vi "Calculate Built Version.vi"(0 "Installer_LV in":refnum<class "Installer_LV.lvclass">, 11 "error in (no error)":errorcluster) -> (4 "Installer_LV out":refnum<class "Installer_LV.lvclass">, 15 "error out":errorcluster)   [LabVIEW 2017, in "CL_G3_VIComponentBuilder.lvlib" / "Installer_LV.lvclass"]
uses:
  Installer_LV.lvclass
  C:/Tool Chain Support/Software Module Builder/Source/Exports/Exports/Export.lvclass
  C:/Tool Chain Support/Software Module Builder/Source/Exports/NI Build Specification_LV/NI Build Specification_LV.lvclass
  Exports/Export.lvclass/Export.ctl
  NI Build Specification_LV/NI Build Specification_LV.lvclass/NI Build Specification_LV.ctl
  Exports/Accessors/Read Exported Build Specification Path.vi
  NI Build Specification_LV/Accessors/Read Build Number XML Prop Name.vi
  Exports/Accessors/Write Built Version.vi
  <vilib>/xml/Load XML File.vi
  <vilib>/xml/Close Reference(Node).vi
  <vilib>/xml/NI_XML.lvlib
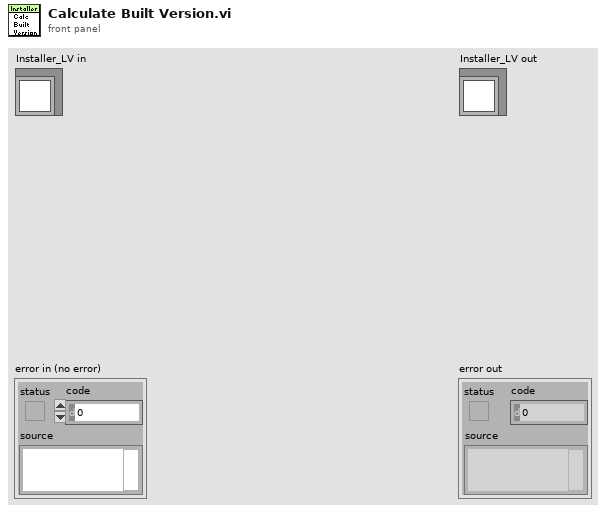
[diagram p1: front panel]
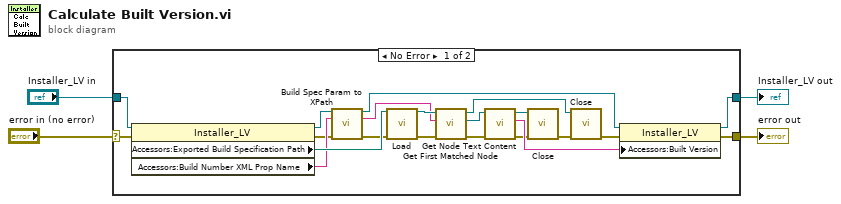
[diagram p0: block diagram]
diagram:
  n1 = case shown="No Error" "error in (no error)" {
    selector: "error in (no error)" -> [w25 w26]
    tunnel: [w15 w26] -> w1
    tunnel: "Installer_LV in" -> [w24 w27]
    tunnel: [w17 w27] -> w2
    frame No Error {
      n2 = property class="Installer_LV"(reference=w24, error in=w25) -> (reference out=w14:refnum<class "Installer_LV.lvclass">, error out=w10:errorcluster, "Accessors:Exported Build Specification Path"=w18:path, "Accessors:Build Number XML Prop Name"=w12:string)
      n3 = call-dynamic "Build Spec Param to XPath.vi"("NI Build Specification"=w14, "Build Spec Parameter Name"=w12, "error in (no error)"=w10) -> ("NI Build Specification"=w13:refnum<class "Installer_LV.lvclass">, "XPath to the specific build Spec Property"=w11:string, "error out"=w9:errorcluster)  [unwired: 10 in]
      n4 = call-poly <vilib>:"Load.vi"("path to XML document"=w18, "error in (no error)"=w9) -> ("DOM document out"=w20:refnum<k20>, "error out"=w19:errorcluster)  [unwired: 11 in, 1 out]
      n5 = call <vilib>:"Get First Matched Node.vi"("error in (no error)"=w19, "XPath expression"=w11, "node in"=w20) -> ("error out"=w22:errorcluster, "node result"=w23:refnum<k20>, "node out"=w21:refnum<k20>)  [unwired: 6 in]
      n6 = call <vilib>:"Get Node Text Content.vi"("error in (no error)"=w22, "node in"=w23) -> ("error out"=w6:errorcluster, "node text"=w8:string, "node out"=w7:refnum<k20>)  [unwired: 7 in]
      n7 = call-poly <vilib>:"Close.vi"("error in (no error)"=w6, "node"=w7) -> ("error out"=w5:errorcluster)  [unwired: 7 in]
      n8 = call-poly <vilib>:"Close.vi"("error in (no error)"=w5, "node"=w21) -> ("error out"=w16:errorcluster)  [unwired: 7 in]
      n9 = property class="Installer_LV"(reference=w13, error in=w16, "Accessors:Built Version"=w8) -> (reference out=w17:refnum<class "Installer_LV.lvclass">, error out=w15:errorcluster)
    }
    frame Error {
    }
  }
  "error out" <- w1
  "Installer_LV out" <- w2
